vi "Euler2Rot.vi"(1 "Ed":dbl[](array[numeric])) -> (0 "Rd":dbl[][](array[numeric]))   [LabVIEW 2018]
uses:
  <vilib>/imath/engines/lvmath2/RunTimeEngine/IndexRead/NIMS V(S).vi
  <instcachedir>/0/NIMS V(S)_0488751826AF41519A22953C041130DC.lvgen/NIMS V(S)_0488751826AF41519A22953C041130DC_000.vi
  <vilib>/imathl/engines/lvmath/Functions/Error Handling/Create Error.vi
  <vilib>/imath/engines/lvmath2/RunTimeEngine/NodeEndStatement/NIMS_NodeEndStatement_Output.vi
  <instcachedir>/0/NIMS_NodeEndStatement_Output_53EC0D466D134D7ABD903AC30B43404B.lvgen/NIMS_NodeEndStatement_Output_53EC0D466D134D7ABD903AC30B43404B_002.vi
  <vilib>/imath/engines/lvmath2/RunTimeEngine/ErrorHandling/NIMS_Finalize Error.vi
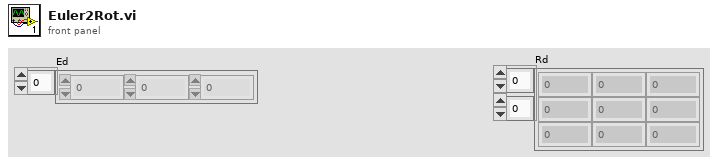
[diagram p1: front panel]
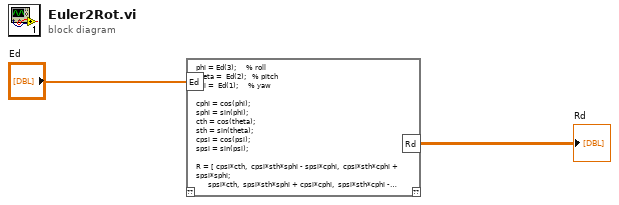
[diagram p0: block diagram]
diagram:
  n1 = mathscript code="phi = Ed(3);     % roll\ntheta =  Ed(2);   % pitch\npsi =  Ed(1);     % yaw\n\ncphi = cos(phi);\nsphi = sin(phi);\ncth = cos(theta);\nsth = sin(theta);\ncpsi = cos(psi);\nspsi = sin(psi);\n\nR = [ cpsi*cth,  cpsi*sth*sphi - spsi*cphi,  cpsi*sth*cphi + spsi*sphi;\n      spsi*cth,  spsi*sth*sphi + cpsi*cphi,  spsi*sth*cphi - cpsi*sphi;\n      -sth,      cth*sphi,                  cth*cphi ];\nRd = R;"("Ed"="Ed") -> ("Rd"=→"Rd":dbl[][])  [unwired: 1 in, 1 out]
